vi "From Single.vi"(4 "CmdAnalog":T2) -> (7 "CmdAnalogMultiple":T1)   [LabVIEW 2023, in "CmdAnalogMultiple.lvlib"]
uses:
  CmdAnalogMultiple.lvlib
  CmdAnalog/Data.ctl
  CmdAnalog/CmdAnalog.lvlib
  Data.ctl
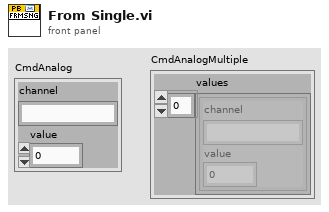
[diagram p1: front panel]
types:
  T1 = typedef "CmdAnalogMultiple.lvlib/Data.ctl" = cluster{"values":T2[]}
  T2 = typedef "CmdAnalog.lvlib/Data.ctl" = cluster{"channel":string, "value":dbl}
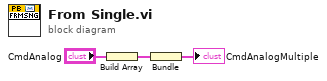
[diagram p0: block diagram]
diagram:
  n1 = Build Array("CmdAnalog") -> (w2:T2[])
  n2 = Bundle(w2) -> (→"CmdAnalogMultiple":cluster{T2[]})  [unwired: 1 in]
